vi "MSCU_Debugger.vi"() -> ()   [LabVIEW 2019]
panel:
  in  "Frequency":i32
  in  "Voltage":i32
  out "Version Code":i32
  in  "Get Version":bool
  in  "Single Step":bool
  out "Status":string="COM Initialized"
  in  "FW/BW":enum32{"Item 0", "Item 1"}(radio)
  in  "Axis":string(combo)
  in  "COM Port":i32
  in  "DLL Path":path
  in  "OK":bool
  # "MSCU \nDebugger"
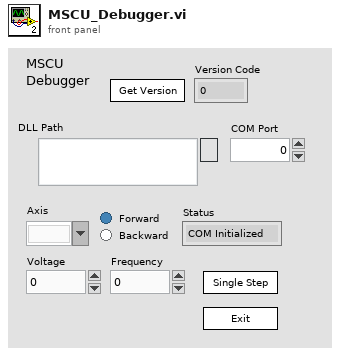
[diagram p1: front panel]
types:
  T1 = enum32{"Invalid", "Standard", "Closed", "Hidden", "Minimized", "Maximized"}
  T2 = enum32{"invalid app kind", "Development System", "Run Time System", "Student Edition", "Embedded LabVIEW", "Evaluation", "Custom"}
  T3 = cluster{"Core":cluster{"Current VI Reference":refnum<vi>, "Close Panel on Exit?":bool}, "DLL Path":path, "COM Port":i32}
  T4 = cluster{"Current VI Reference":refnum<vi>, "Close Panel on Exit?":bool}
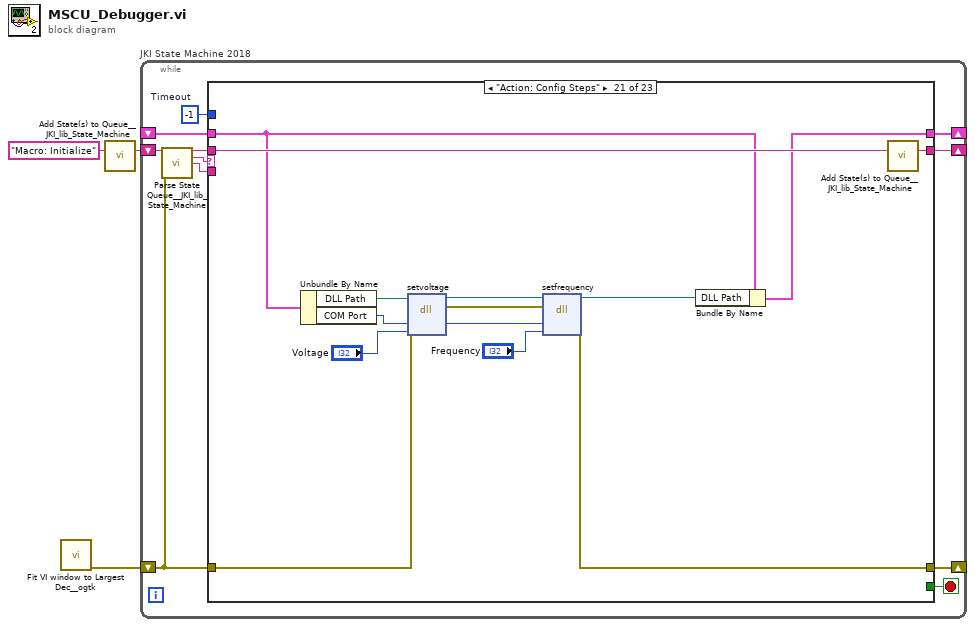
[diagram p0: block diagram]
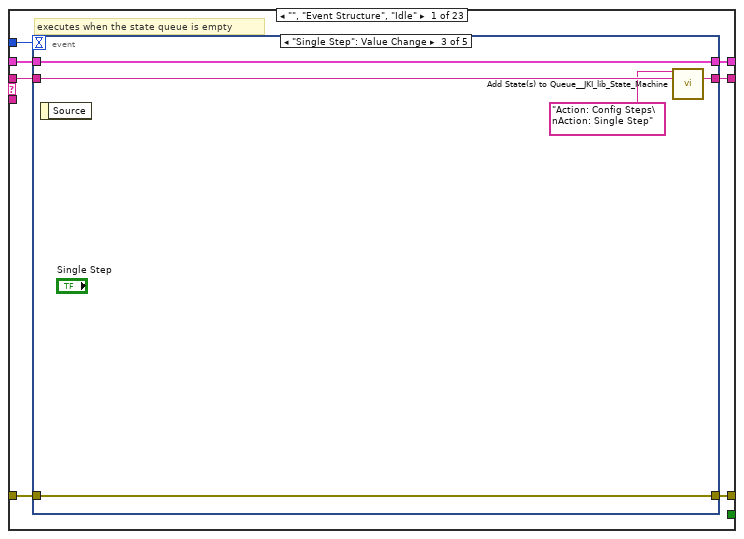
[diagram p2: hidden frame]
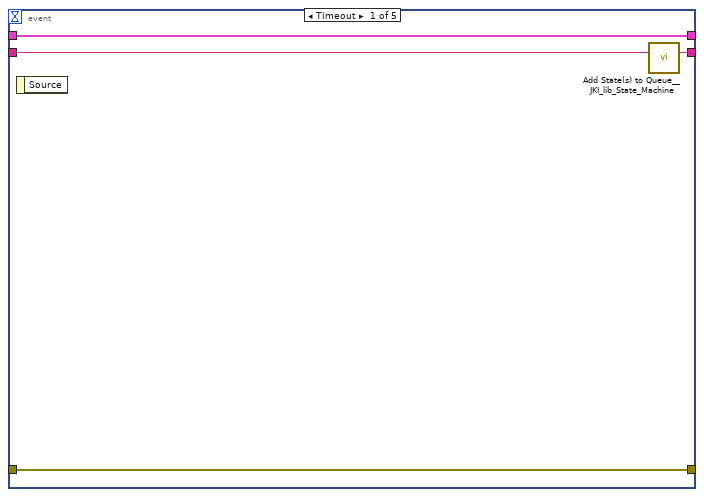
[diagram p3: hidden frame]
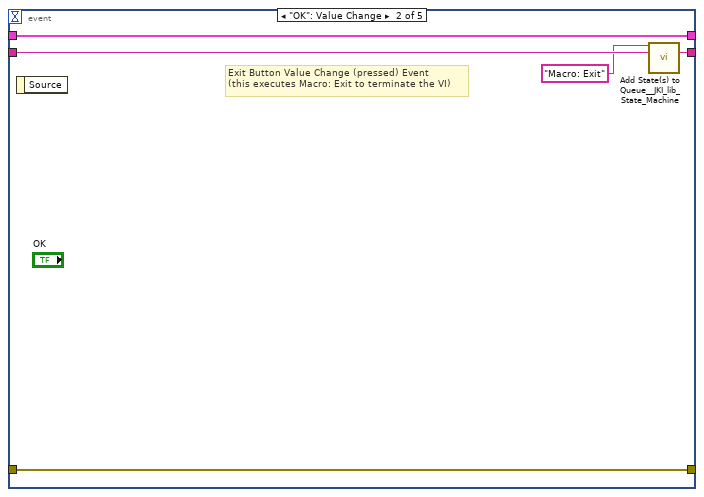
[diagram p4: hidden frame]
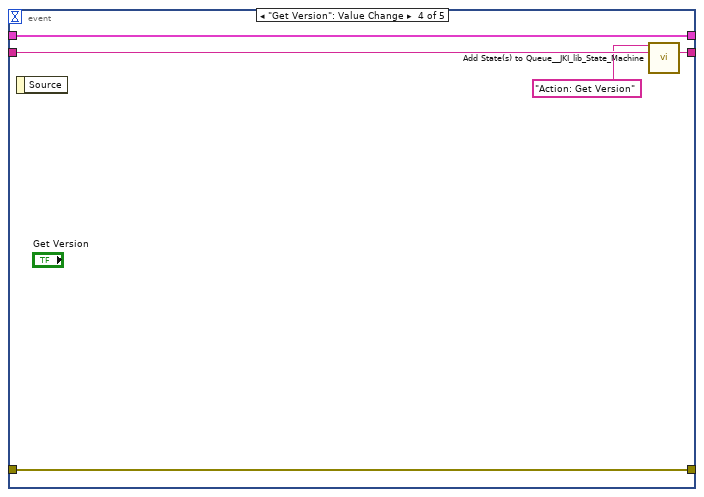
[diagram p5: hidden frame]
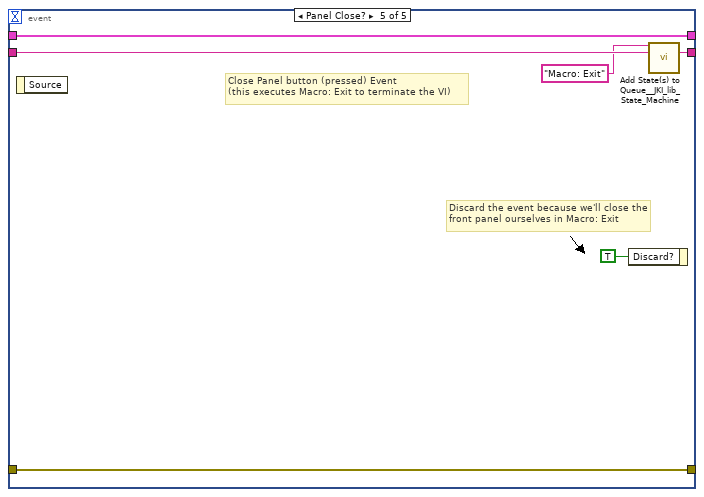
[diagram p6: hidden frame]
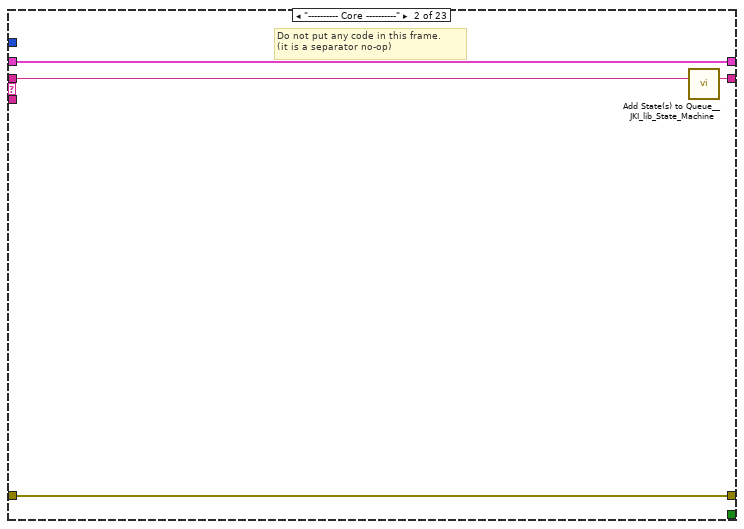
[diagram p7: hidden frame]
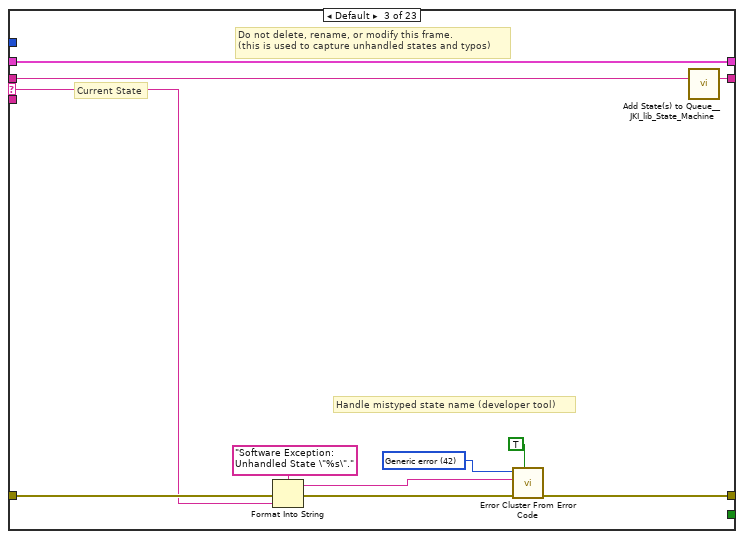
[diagram p8: hidden frame]
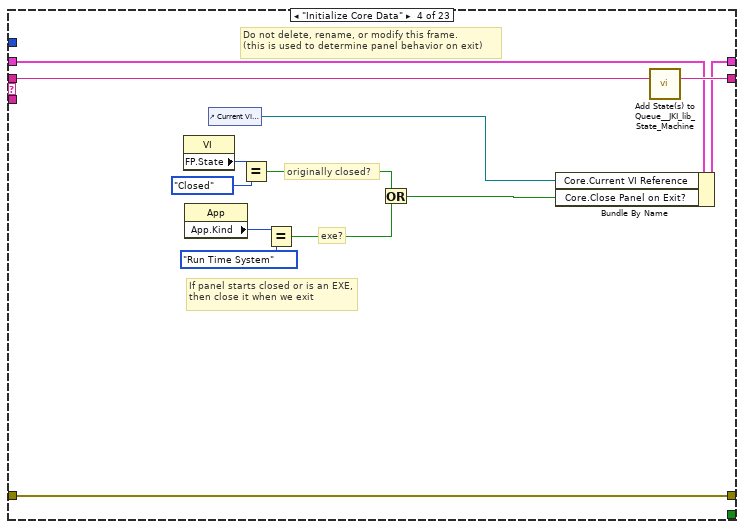
[diagram p9: hidden frame]
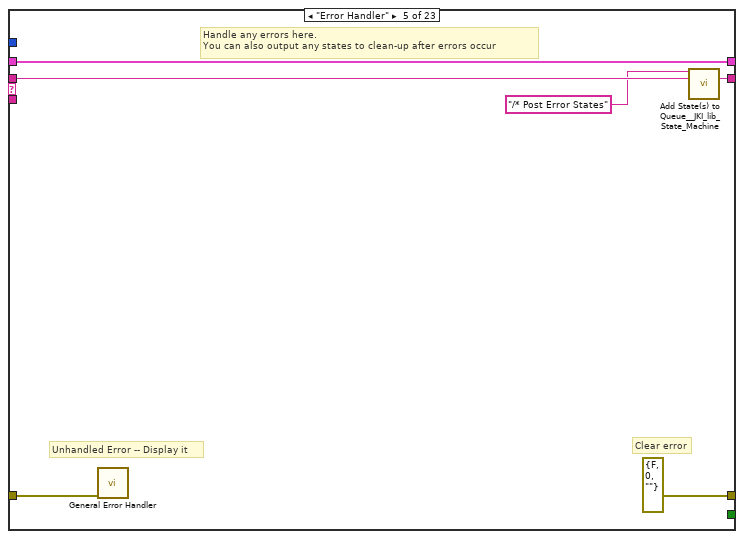
[diagram p10: hidden frame]
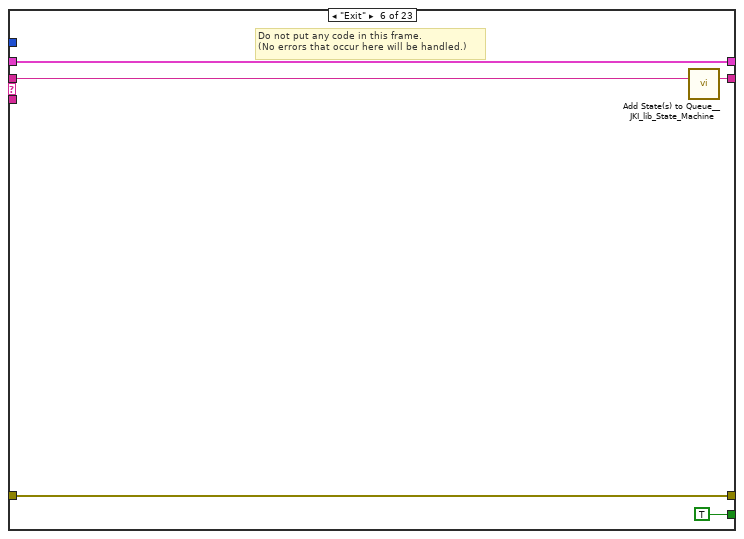
[diagram p11: hidden frame]
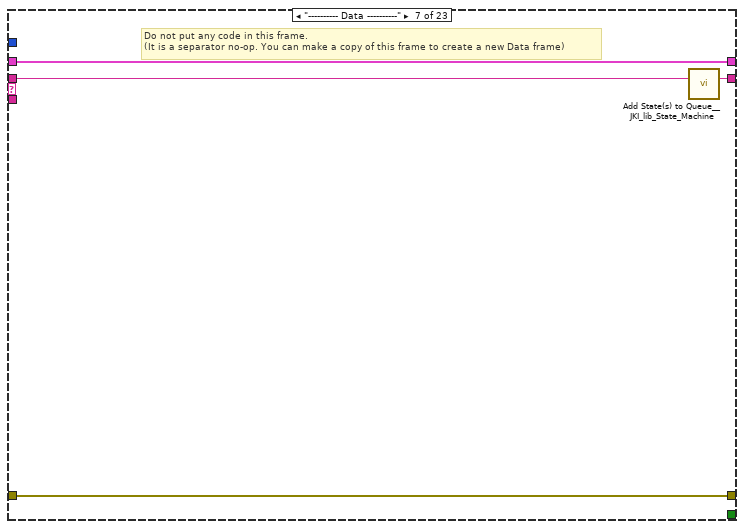
[diagram p12: hidden frame]
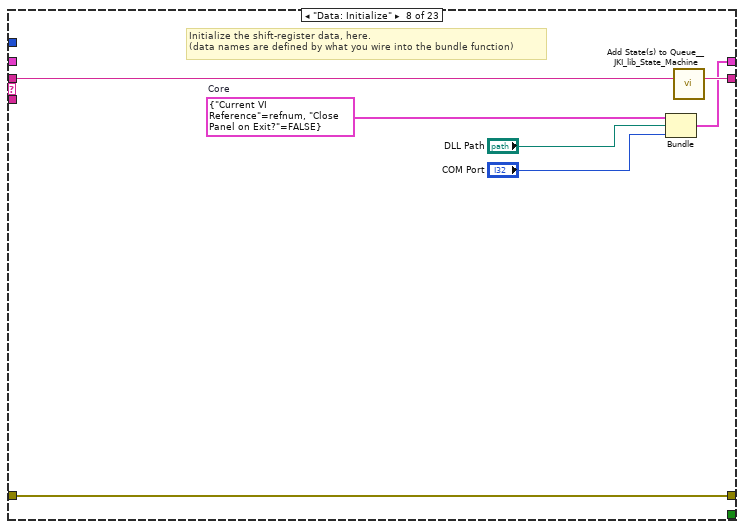
[diagram p13: hidden frame]
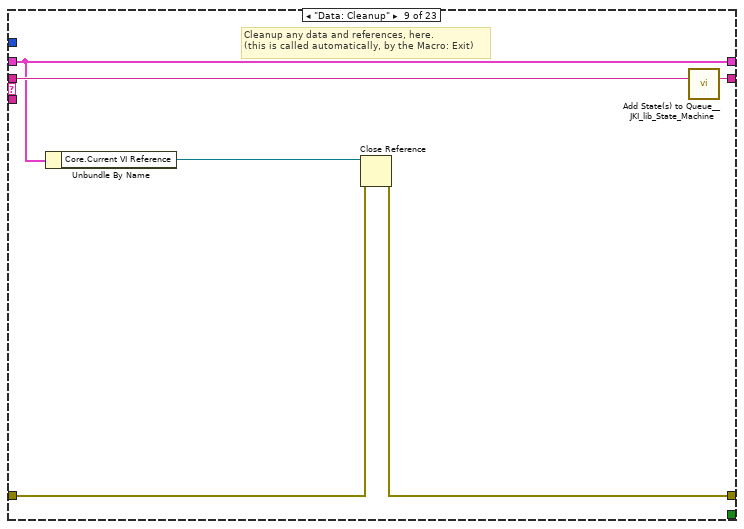
[diagram p14: hidden frame]
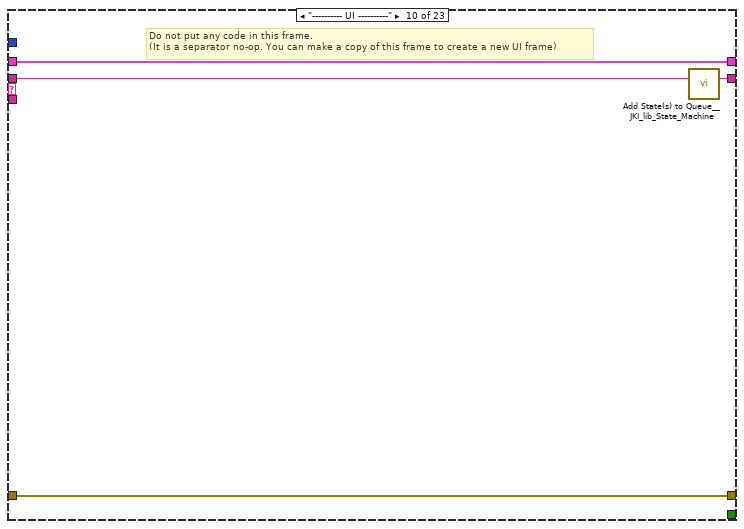
[diagram p15: hidden frame]
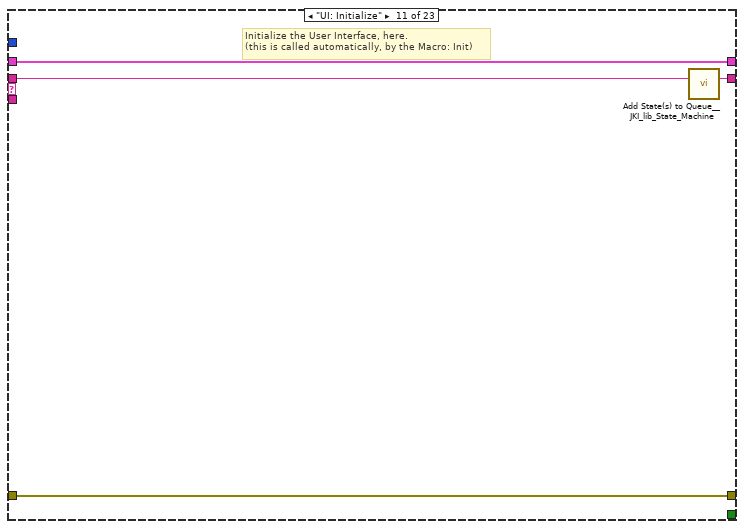
[diagram p16: hidden frame]
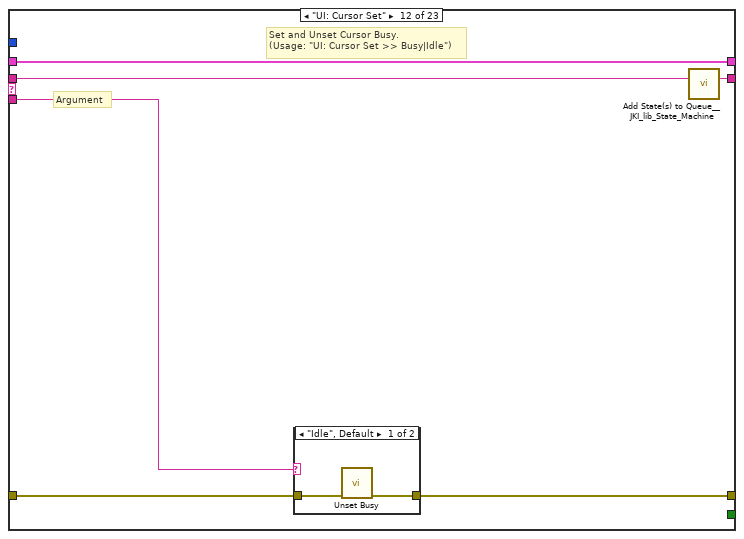
[diagram p17: hidden frame]
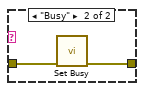
[diagram p18: hidden frame]
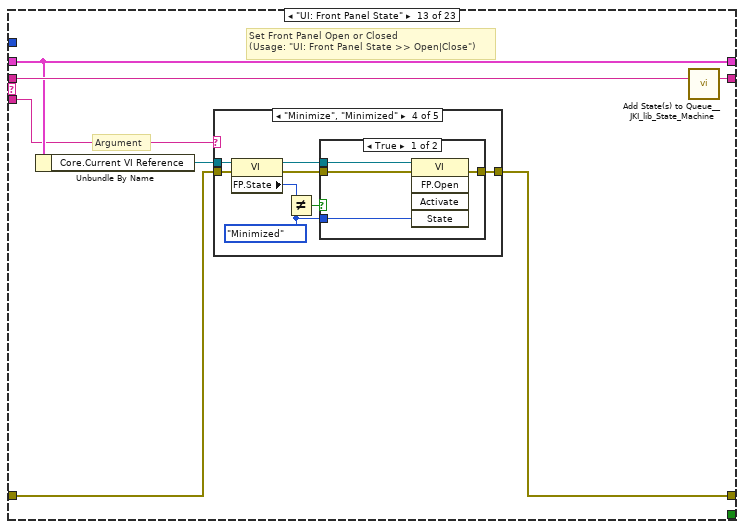
[diagram p19: hidden frame]
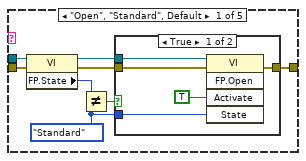
[diagram p20: hidden frame]
diagram:
  n1 = call <userlib>:"Fit VI window to Largest Dec__ogtk.vi"() -> ("error out"=w1:errorcluster)  [unwired: 6 in, 1 out]
  n2 = call <vilib>:"Add State(s) to Queue__JKI_lib_State_Machine.vi"("State(s) in (\"\")"="Macro: Initialize") -> ("States Out"=w3:string)  [unwired: 14 in]
  n3 = while "JKI State Machine 2018" {
    shift-right: [w7] -> _
    shift-left: _ -> [w6]
    shift-right: [w10] -> _
    shift-left: w1 -> [w4]
    shift-right: [w9] -> _
    shift-left: w3 -> [w11]
    stop <- w8 stop-if-true
    w5 = -1  # Timeout
    n4 = call <vilib>:"Parse State Queue__JKI_lib_State_Machine.vi"("State Queue"=w11, "Error In (no error)"=w4) -> ("Remaining States"=w13:string, "Current State"=w14:string, "Arguments"=w12:string)  [unwired: 11 in]
    n5 = case shown="\"Action: Config Steps\"" w14 {
      selector: w14 -> [_ _ w51 _ _ _ _ _ _ _ _ _ _ _ _ _ _ _ _ _ _ _ _]
      tunnel: w13 -> [w21 w50 w55 w74 w80 w85 w89 w96 w102 w106 w110 w116 w127 w196 w201 w211 w215 w226 w239 w248 w262 w275 w290]
      tunnel: w12 -> [_ _ _ _ _ _ _ _ _ _ _ w111 w121 _ _ _ _ _ _ _ _ _ _]
      tunnel: w6 -> [w19 w47 w53 w67 w77 w83 w86 _ w97 w103 w108 w114 w123 w193 w198 w208 w212 w224 w237 w242 w260 w273 w288]
      tunnel: [w18 w48 w57 w71 errorcluster {"status"=FALSE, "code"=0, "source"=""} ("error out") w82 w87 w93 w98 w104 w107 w112 w124 w194 w199 w209 w213 w220 w234 w245 w253 w267 w283] -> w10
      tunnel: w4 -> [w17 w48 w56 w71 w76 w82 w87 w93 w99 w104 w107 w113 w125 w194 w199 w209 w213 w219 w235 w246 w254 w268 w284]
      tunnel: [w20 w49 w54 w73 w79 w84 w88 w95 w101 w105 w109 w115 w126 w195 w200 w210 w214 w225 w238 w247 w261 w274 w289] -> w9
      tunnel: [_ _ _ _ _ TRUE _ _ _ _ _ _ _ _ _ _ _ _ _ _ _ _ _] -> w8
      tunnel: [w16 w47 w53 w72 w77 w83 w86 w94 w97 w103 w108 w114 w123 w193 w198 w208 w212 w223 w236 w241 w259 w272 w287] -> w7
      tunnel: w5 -> [w15 _ _ _ _ _ _ _ _ _ _ _ _ _ _ _ _ _ _ _ _ _ _]
      frame "", "Event Structure", "Idle" {
        # "executes when the state queue is empty"
        n6 = event shown="[2] \"Single Step\": Value Change" {
          selector: _ -> [_ _ _ _ _]
          dyn-events: _ -> [_ _ _ _ _]
          timeout: w15 -> [_ _ _ _ _]
          tunnel: w21 -> [w25 w30 w35 w40 w46]
          tunnel: [w24 w29 w34 w39 w45] -> w20
          tunnel: w19 -> [w22 w27 w32 w37 w43]
          tunnel: [w23 w28 w33 w38 w44] -> w18
          tunnel: w17 -> [w23 w28 w33 w38 w44]
          tunnel: [w22 w27 w32 w37 w43] -> w16
          event Timeout {
            n7 = event-data() -> ()  [unwired: 1 in, 1 out]
            n8 = call <vilib>:"Add State(s) to Queue__JKI_lib_State_Machine.vi"("State(s) in (\"\")"=w25) -> ("States Out"=w24:string)  [unwired: 14 in]
          }
          event "OK": Value Change {
            # "Exit Button Value Change (pressed) Event\n(this executes Macro: Exit to terminate the VI)"
            n9 = event-data() -> ()  [unwired: 1 in, 1 out]
            n10 = call <vilib>:"Add State(s) to Queue__JKI_lib_State_Machine.vi"("State(s) in Front (\"\")"="Macro: Exit", "State(s) in (\"\")"=w30) -> ("States Out"=w29:string)  [unwired: 13 in]
          }
          event "Single Step": Value Change {
            n11 = event-data() -> ()  [unwired: 1 in, 1 out]
            n12 = call <vilib>:"Add State(s) to Queue__JKI_lib_State_Machine.vi"("State(s) in Front (\"\")"="Action: Config Steps\nAction: Single Step", "State(s) in (\"\")"=w35) -> ("States Out"=w34:string)  [unwired: 13 in]
          }
          event "Get Version": Value Change {
            n13 = event-data() -> ()  [unwired: 1 in, 1 out]
            n14 = call <vilib>:"Add State(s) to Queue__JKI_lib_State_Machine.vi"("State(s) in Front (\"\")"="Action: Get Version", "State(s) in (\"\")"=w40) -> ("States Out"=w39:string)  [unwired: 13 in]
          }
          event Panel Close? {
            # "Discard the event because we'll close the front panel ourselves in Macro: Exit"
            # "Close Panel button (pressed) Event\n(this executes Macro: Exit to terminate the VI)"
            n15 = event-data() -> ()  [unwired: 1 in, 1 out]
            n16 = event-data("Discard?"=TRUE) -> ()  [unwired: 1 in, 1 out]
            n17 = call <vilib>:"Add State(s) to Queue__JKI_lib_State_Machine.vi"("State(s) in Front (\"\")"="Macro: Exit", "State(s) in (\"\")"=w46) -> ("States Out"=w45:string)  [unwired: 13 in]
          }
        }
      }
      frame "---------- Core ----------" {
        # "Do not put any code in this frame.\n(it is a separator no-op)"
        n18 = call <vilib>:"Add State(s) to Queue__JKI_lib_State_Machine.vi"("State(s) in (\"\")"=w50) -> ("States Out"=w49:string)  [unwired: 14 in]
      }
      frame Default {
        w60 = 42 items=["No error", "Argument error", "Memory is full", "Out of zone", "End of file", "File already open", "Generic file I/O error", "File not found", "File permission error", "Disk is full", "Duplicate path", "Too many files open", "System feature not enabled", "Resource file not found", "Cannot add resource", "Resource not found", "Image not found", "Image memory error", "Pen does not exist", "Config type invalid", "Config token not found", "Config parse error", "Config memory error", "Bad external code format", "Bad external code offset", "External code not present", "Null window", "Destroy window error", "Null menu", "Print aborted", "Bad print record", "Print driver error", "Windows error during printing", "Memory error during printing", "Print dialog error", "Generic print error", "Invalid device refnum", "Device not found", "Device parameter error", "Device unit error", "Cannot open device", "Device call aborted", "Generic error", "Cancelled by user", "Object ID too low", "Object ID too high", "Object not in heap", "Unknown heap", "Unknown object (invalid DefProc)", "Unknown object (DefProc not in table)", "Message out of range", "Invalid (null) method", "Unknown message", "Manager call not supported", "Bad address", "Network operation in progress", "Network operation timed out", "Connection is busy", "Network attribute not supported", "Network error", "Address in use", "System out of memory", "Connection aborted", "Connection refused", "Not connected", "Already connected", "Connection closed", "Initialization error (interapplication manager)", "Bad occurrence", "Wait on unbound occurrence handler", "Occurrence queue overflow", "Datalog type conflict", "Unused", "Unrecognized type (interapplication manager)", "Memory corrupt", "Failed to make temporary DLL", "Old CIN version", "Drag socket not found", "Failed to load drop-object", "Failed to register OLE object", "Failed to release OLE object", "Format specifier type mismatch", "Unknown format specifier", "Too few format specifiers", "Too many format specifiers", "Scan failed", "Newer CIN version", "Error converting to variant", "Runtime menu error", "Password tampered", "Variant attribute not found", "Incompatible variant data type", "Event data is not available", "Event Store is not present", "Occurrence is not found", "Event Queue is not created", "Event info is not available", "Refnum passed is NULL", "Error retrieving Class GUID", "Error retrieving CoClass GUID", "Error retrieving TypeLib GUID.", "Bad built application magic bytes.", "Specific driver is different from the specific driver associated with the Logical Name.", "There is no session opened to the class driver.", "Max Error", "MAX - Error with config objects", "MAX - Error loading configuration", "MAX - Group not supported"]
        # "Current State"
        # "Do not delete, rename, or modify this frame.\n(this is used to capture unhandled states and typos)"
        # "Handle mistyped state name (developer tool)"
        n19 = Format Into String(format string="Software Exception: Unhandled State \"%s\"." ("message"), error in=w56, w51) -> (resulting string=w59:string, error out=w58:errorcluster)  [unwired: 1 in]
        n20 = call <vilib>:"Error Cluster From Error Code.vi"("show call chain? (False)"=TRUE, "error in (no error)"=w58, "error message (\"\")"=w59, "error code (0)"=w60) -> ("error out"=w57:errorcluster)  [unwired: 5 in]
        n21 = call <vilib>:"Add State(s) to Queue__JKI_lib_State_Machine.vi"("State(s) in (\"\")"=w55) -> ("States Out"=w54:string)  [unwired: 14 in]
      }
      frame "Initialize Core Data" {
        # "Do not delete, rename, or modify this frame.\n(this is used to determine panel behavior on exit)"
        # "originally closed?"
        # "exe?"
        # "If panel starts closed or is an EXE, then close it when we exit"
        n22 = property class="VI"() -> ("FP.State"=w64:T1)  [unwired: 2 in, 2 out]
        n23 = property class="App"() -> ("App.Kind"=w70:T2)  [unwired: 2 in, 2 out]
        n24 = control-ref of="Current VI Reference"() -> (w65:refnum<vi>)
        n25 = Equal?(x=w64, y=T1."Closed" ("Front Panel Window:State")) -> (x = y?=w62:bool)
        n26 = Equal?(x=w70, y=T2."Run Time System" ("Application:Kind")) -> (x = y?=w68:bool)
        n27 = Or(x=w62, y=w68) -> (x .or. y?=w66:bool)
        n28 = Bundle By Name(cluster=w67, "Core.Current VI Reference"=w65, "Core.Close Panel on Exit?"=w66) -> (w72:T3)
        n29 = call <vilib>:"Add State(s) to Queue__JKI_lib_State_Machine.vi"("State(s) in (\"\")"=w74) -> ("States Out"=w73:string)  [unwired: 14 in]
      }
      frame "Error Handler" {
        # "Unhandled Error -- Display it"
        # "Handle any errors here.\nYou can also output any states to clean-up after errors occur"
        # "Clear error"
        n30 = call <vilib>:"General Error Handler.vi"("error in (no error)"=w76) -> ()  [unwired: 10 in, 5 out]
        n31 = call <vilib>:"Add State(s) to Queue__JKI_lib_State_Machine.vi"("State(s) in Front (\"\")"="/* Post Error States", "State(s) in (\"\")"=w80) -> ("States Out"=w79:string)  [unwired: 13 in]
      }
      frame "Exit" {
        # "Do not put any code in this frame.\n(No errors that occur here will be handled.)"
        n32 = call <vilib>:"Add State(s) to Queue__JKI_lib_State_Machine.vi"("State(s) in (\"\")"=w85) -> ("States Out"=w84:string)  [unwired: 14 in]
      }
      frame "---------- Data ----------" {
        # "Do not put any code in this frame.\n(It is a separator no-op. You can make a copy of this frame to create a new Data frame)"
        n33 = call <vilib>:"Add State(s) to Queue__JKI_lib_State_Machine.vi"("State(s) in (\"\")"=w89) -> ("States Out"=w88:string)  [unwired: 14 in]
      }
      frame "Data: Initialize" {
        w92 = T4 {"Current VI Reference"=refnum, "Close Panel on Exit?"=FALSE}  # Core
        # "Initialize the shift-register data, here.\n(data names are defined by what you wire into the bundle function)"
        n34 = Bundle("Core"=w92, "DLL Path"="DLL Path", "COM Port"="COM Port") -> (w94:T3)  [unwired: 1 in]
        n35 = call <vilib>:"Add State(s) to Queue__JKI_lib_State_Machine.vi"("State(s) in (\"\")"=w96) -> ("States Out"=w95:string)  [unwired: 14 in]
      }
      frame "Data: Cleanup" {
        # "Cleanup any data and references, here.\n(this is called automatically, by the Macro: Exit)"
        n36 = Unbundle By Name(w97) -> ("Core.Current VI Reference"=w100:refnum<vi>)
        n37 = Close Reference(reference=w100, error in (no error)=w99) -> (error out=w98:errorcluster)
        n38 = call <vilib>:"Add State(s) to Queue__JKI_lib_State_Machine.vi"("State(s) in (\"\")"=w102) -> ("States Out"=w101:string)  [unwired: 14 in]
      }
      frame "---------- UI ----------" {
        # "Do not put any code in this frame.\n(It is a separator no-op. You can make a copy of this frame to create a new UI frame)"
        n39 = call <vilib>:"Add State(s) to Queue__JKI_lib_State_Machine.vi"("State(s) in (\"\")"=w106) -> ("States Out"=w105:string)  [unwired: 14 in]
      }
      frame "UI: Initialize" {
        # "Initialize the User Interface, here.\n(this is called automatically, by the Macro: Init)"
        n40 = call <vilib>:"Add State(s) to Queue__JKI_lib_State_Machine.vi"("State(s) in (\"\")"=w110) -> ("States Out"=w109:string)  [unwired: 14 in]
      }
      frame "UI: Cursor Set" {
        # "Argument"
        # "Set and Unset Cursor Busy.\n(Usage: \"UI: Cursor Set >> Busy|Idle\")"
        n41 = case shown="\"Idle\", Default" w111 {
          tunnel: w113 -> [w118 w120]
          tunnel: [w117 w119] -> w112
          frame "Idle", Default {
            n42 = call <vilib>:"Unset Busy.vi"("error in (no error)"=w118) -> ("error out"=w117:errorcluster)  [unwired: 10 in]
          }
          frame "Busy" {
            n43 = call <vilib>:"Set Busy.vi"("error in (no error)"=w120) -> ("error out"=w119:errorcluster)  [unwired: 9 in, 1 out]
          }
        }
        n44 = call <vilib>:"Add State(s) to Queue__JKI_lib_State_Machine.vi"("State(s) in (\"\")"=w116) -> ("States Out"=w115:string)  [unwired: 14 in]
      }
      frame "UI: Front Panel State" {
        # "Argument"
        # "Set Front Panel Open or Closed\n(Usage: \"UI: Front Panel State >> Open|Close\")"
        n45 = Unbundle By Name(w123) -> ("Core.Current VI Reference"=w122:refnum<vi>)
        n46 = case shown="\"Minimize\", \"Minimized\"" w121 {
          tunnel: w125 -> [w133 w148 w159 w172 w185]
          tunnel: [w135 w149 w161 w174 w187] -> w124
          tunnel: w122 -> [w134 w146 w160 w173 w186]
          frame "Open", "Standard", Default {
            w128 = T1."Standard" ("State")
            n47 = property class="VI"(reference=w134, error in=w133) -> (reference out=w131:refnum<vi>, error out=w132:errorcluster, "FP.State"=w130:T1)
            n48 = Not Equal?(x=w130, y=w128) -> (x != y?=w129:bool)
            n49 = case shown="True" w129 {
              tunnel: [w139 w141] -> w135
              tunnel: w132 -> [w138 w141]
              tunnel: w131 -> [w137 _]
              tunnel: w128 -> [w136 _]
              frame True {
                n50 = invoke class="VI" method="FP.Open"(reference=w137, error in=w138, "Activate"=TRUE, "State"=w136) -> (error out=w139:errorcluster)  [unwired: 1 in, 4 out]
              }
              frame False {
              }
            }
          }
          frame "Close", "Closed" {
            n51 = property class="VI"(reference=w146, error in=w148) -> (reference out=w145:refnum<vi>, error out=w147:errorcluster, "FP.State"=w143:T1)
            n52 = Not Equal?(x=w143, y=T1."Closed" ("Front Panel Window:State")) -> (x != y?=w142:bool)
            n53 = case shown="True" w142 {
              tunnel: [w150 w153] -> w149
              tunnel: w147 -> [w150 w152]
              tunnel: w145 -> [_ w151]
              frame False {
              }
              frame True {
                n54 = invoke class="VI" method="FP.Close"(reference=w151, error in=w152) -> (error out=w153:errorcluster)  [unwired: 1 in, 2 out]
              }
            }
          }
          frame "Hidden", "Hide" {
            w154 = T1."Hidden" ("State")
            n55 = property class="VI"(reference=w160, error in=w159) -> (reference out=w157:refnum<vi>, error out=w158:errorcluster, "FP.State"=w156:T1)
            n56 = Not Equal?(x=w156, y=w154) -> (x != y?=w155:bool)
            n57 = case shown="True" w155 {
              tunnel: [w165 w166] -> w161
              tunnel: w158 -> [w164 w166]
              tunnel: w157 -> [w163 _]
              tunnel: w154 -> [w162 _]
              frame True {
                n58 = invoke class="VI" method="FP.Open"(reference=w163, error in=w164, "State"=w162) -> (error out=w165:errorcluster)  [unwired: 2 in, 4 out]
              }
              frame False {
              }
            }
          }
          frame "Minimize", "Minimized" {
            w167 = T1."Minimized" ("State")
            n59 = property class="VI"(reference=w173, error in=w172) -> (reference out=w170:refnum<vi>, error out=w171:errorcluster, "FP.State"=w169:T1)
            n60 = Not Equal?(x=w169, y=w167) -> (x != y?=w168:bool)
            n61 = case shown="True" w168 {
              tunnel: [w178 w179] -> w174
              tunnel: w171 -> [w177 w179]
              tunnel: w170 -> [w176 _]
              tunnel: w167 -> [w175 _]
              frame True {
                n62 = invoke class="VI" method="FP.Open"(reference=w176, error in=w177, "State"=w175) -> (error out=w178:errorcluster)  [unwired: 2 in, 4 out]
              }
              frame False {
              }
            }
          }
          frame "Maximize", "Maximized" {
            w180 = T1."Maximized" ("State")
            n63 = property class="VI"(reference=w186, error in=w185) -> (reference out=w183:refnum<vi>, error out=w184:errorcluster, "FP.State"=w182:T1)
            n64 = Not Equal?(x=w182, y=w180) -> (x != y?=w181:bool)
            n65 = case shown="True" w181 {
              tunnel: [w191 w192] -> w187
              tunnel: w184 -> [w190 w192]
              tunnel: w183 -> [w189 _]
              tunnel: w180 -> [w188 _]
              frame True {
                n66 = invoke class="VI" method="FP.Open"(reference=w189, error in=w190, "State"=w188) -> (error out=w191:errorcluster)  [unwired: 2 in, 4 out]
              }
              frame False {
              }
            }
          }
        }
        n67 = call <vilib>:"Add State(s) to Queue__JKI_lib_State_Machine.vi"("State(s) in (\"\")"=w127) -> ("States Out"=w126:string)  [unwired: 14 in]
      }
      frame "---------- Macro ----------" {
        # "Do not put any code in this frame.\n(It is a separator no-op. You can make a copy of this frame to create a new Macro frame)"
        n68 = call <vilib>:"Add State(s) to Queue__JKI_lib_State_Machine.vi"("State(s) in (\"\")"=w196) -> ("States Out"=w195:string)  [unwired: 14 in]
      }
      frame "Macro: Initialize" {
        w197 = "Data: Initialize\nInitialize Core Data\nUI: Initialize\nUI: Front Panel State >> Open\nAction: Init COM"  # Data: Initialize Initialize Core Data UI: Initialize UI: Front Panel State >> Open Action: Init COM
        # "Initialization Macro\n(This is called once, when the VI starts)"
        n69 = call <vilib>:"Add State(s) to Queue__JKI_lib_State_Machine.vi"("State(s) in Front (\"\")"=w197, "State(s) in (\"\")"=w201) -> ("States Out"=w200:string)  [unwired: 13 in]
      }
      frame "Macro: Exit" {
        # "Exit Macro\n(This is called once, when the VI exits)"
        n70 = Unbundle By Name(w208) -> ("Core.Close Panel on Exit?"=w207:bool)
        n71 = Select(t="UI: Front Panel State >> Close", s=w207, f="") -> (s? t:f=w204:string)
        n72 = call <vilib>:"Add State(s) to Queue__JKI_lib_State_Machine.vi"("State(s) in (\"\")"=w204, "State(s) at Back (\"\")"="Action: Init COM\nData: Cleanup\nExit") -> ("States Out"=w202:string)  [unwired: 13 in]
        n73 = call <vilib>:"Add State(s) to Queue__JKI_lib_State_Machine.vi"("State(s) in Front (\"\")"=w202, "State(s) in (\"\")"=w211) -> ("States Out"=w210:string)  [unwired: 13 in]
      }
      frame "---------- Action ----------" {
        # "Template Separator\n(You can make a copy of, or modify, this frame)"
        n74 = call <vilib>:"Add State(s) to Queue__JKI_lib_State_Machine.vi"("State(s) in (\"\")"=w215) -> ("States Out"=w214:string)  [unwired: 14 in]
      }
      frame "Action: Init COM" {
        # "-1 should be assigned for an error.\nI'm just using this for 'COM closed' until I fix Close COM"
        n75 = Unbundle By Name(w224) -> ("DLL Path"=w222:path, "COM Port"=w218:i32)
        n76 = dll-call lib="C:/Program Files (x86)/Nanonis/SPM Controller/data/MSCU.dll" fn="configcom"(path in=w222, error in=w219, "Comport"=w218) -> (path out=w221:path, error out=w220:errorcluster, "return type"=w217:i32)  [unwired: 2 in]
        n77 = case shown="1, Default" w217 {
          tunnel: ["COM Initialized" "COM Closed"] -> w216
          frame 1, Default {
          }
          frame -1 {
          }
        }
        "Status" <- w216
        n78 = Bundle By Name(cluster=w224, "DLL Path"=w221) -> (w223:T3)
        n79 = call <vilib>:"Add State(s) to Queue__JKI_lib_State_Machine.vi"("State(s) in (\"\")"=w226) -> ("States Out"=w225:string)  [unwired: 14 in]
      }
      frame "Action: Close COM" {
        # "Currently not working.\nThere was an issue with Closing the COM port\nShould address later"
        n80 = Unbundle By Name(w237) -> ("COM Port"=w232:i32)
        n81 = Number To Decimal String(number=w232) -> (decimal integer string=w231:string)  [unwired: 1 in]
        n82 = Concatenate Strings("COM" ("string"), w231) -> (w230:string)
        n83 = VISA Close(VISA resource name=w230, error in (no error)=w235) -> (error out=w234:errorcluster)
        n84 = Bundle By Name(cluster=w237, "DLL Path"=path "") -> (w236:T3)
        n85 = call <vilib>:"Add State(s) to Queue__JKI_lib_State_Machine.vi"("State(s) in (\"\")"=w239) -> ("States Out"=w238:string)  [unwired: 14 in]
      }
      frame "Action: Get Status" {
        n86 = Unbundle By Name(w242) -> ("DLL Path"=w244:path, "COM Port"=w243:i32)
        n87 = dll-call lib="C:/Program Files (x86)/Nanonis/SPM Controller/data/MSCU.dll" fn="getstatus"(path in=w244, error in=w246, "Comport"=w243) -> (path out=w240:path, error out=w245:errorcluster)  [unwired: 3 in]
        n88 = Bundle By Name(cluster=w242, "DLL Path"=w240) -> (w241:T3)
        n89 = call <vilib>:"Add State(s) to Queue__JKI_lib_State_Machine.vi"("State(s) in (\"\")"=w248) -> ("States Out"=w247:string)  [unwired: 14 in]
      }
      frame "Action: Config Steps" {
        n90 = Unbundle By Name(w260) -> ("DLL Path"=w258:path, "COM Port"=w251:i32)
        n91 = dll-call lib="C:/Program Files (x86)/Nanonis/SPM Controller/data/MSCU.dll" fn="setvoltage"(path in=w258, error in=w254, "Comport"=w251, "Voltage"="Voltage") -> (path out=w256:path, error out=w255:errorcluster, "Comport"=w252:i32)  [unwired: 3 in]
        n92 = dll-call lib="C:/Program Files (x86)/Nanonis/SPM Controller/data/MSCU.dll" fn="setfrequency"(path in=w256, error in=w255, "Comport"=w252, "Frequency"="Frequency") -> (path out=w257:path, error out=w253:errorcluster)  [unwired: 4 in]
        n93 = Bundle By Name(cluster=w260, "DLL Path"=w257) -> (w259:T3)
        n94 = call <vilib>:"Add State(s) to Queue__JKI_lib_State_Machine.vi"("State(s) in (\"\")"=w262) -> ("States Out"=w261:string)  [unwired: 14 in]
      }
      frame "Action: Single Step" {
        n95 = Unbundle By Name(w273) -> ("DLL Path"=w271:path, "COM Port"=w269:i32)
        n96 = case shown="\"z\"" "Axis" {
          tunnel: [1 2 3] -> w265
          frame "x", Default {
          }
          frame "y" {
          }
          frame "z" {
          }
        }
        n97 = case shown="\"Item 0\", Default" "FW/BW" {
          tunnel: [-1 1] -> w264
          frame "Item 0", Default {
          }
          frame "Item 1" {
          }
        }
        n98 = dll-call lib="C:/Program Files (x86)/Nanonis/SPM Controller/data/MSCU.dll" fn="singlestep"(path in=w271, error in=w268, "Comport"=w269, "Channel"=w265, "Direction"=w264) -> (path out=w270:path, error out=w267:errorcluster)  [unwired: 5 in]
        n99 = Bundle By Name(cluster=w273, "DLL Path"=w270) -> (w272:T3)
        n100 = call <vilib>:"Add State(s) to Queue__JKI_lib_State_Machine.vi"("State(s) in (\"\")"=w275) -> ("States Out"=w274:string)  [unwired: 14 in]
      }
      frame "Action: Get Version" {
        n101 = Unbundle By Name(w288) -> ("DLL Path"=w286:path, "COM Port"=w285:i32)
        n102 = dll-call lib="C:/Program Files (x86)/Nanonis/SPM Controller/data/MSCU.dll" fn="getversion"(path in=w286, error in=w284, "Comport"=w285) -> (path out=w282:path, error out=w283:errorcluster, "return type"=→"Version Code":i32)  [unwired: 2 in]
        n103 = Bundle By Name(cluster=w288, "DLL Path"=w282) -> (w287:T3)
        n104 = call <vilib>:"Add State(s) to Queue__JKI_lib_State_Machine.vi"("State(s) in (\"\")"=w290) -> ("States Out"=w289:string)  [unwired: 14 in]
      }
    }
  }
